vi "Read Map - Row.vi"(10 "Row":i32, 11 "map":refnum<data-value>) -> (2 "square states":T1[](array[typedef]), 3 "map":refnum<data-value>)   [LabVIEW 2020, in "DS Square.lvlib"]
uses:
  DS Square.lvlib
  Map.ctl
  Square Status.ctl
  Square State.ctl
  Center of Mass.ctl
  SubVIs/Read-Only Globals.vi
  SubVIs/Globals (private).vi
  Square/Square.lvclass
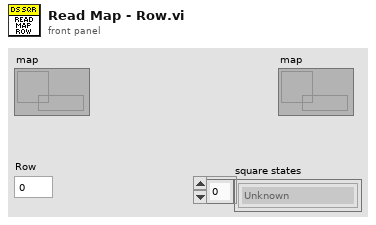
[diagram p1: front panel]
types:
  T1 = typedef "DS Square.lvlib/Square State.ctl" = enum16{"Unknown", "Empty", "Occupied - Active", "Occupied - Cool Down", "Attacked", "Enemy", "Enemy Wall"}
  T2 = typedef "DS Square.lvlib/Map.ctl" = cluster{"squares":T3[][], "center of mass":T4}
  T3 = typedef "DS Square.lvlib/Square Status.ctl" = cluster{"square state":T1, "probability":dbl, "last update":i32}
  T4 = typedef "DS Square.lvlib/Center of Mass.ctl" = cluster{"row":dbl, "col":dbl, "mass":dbl}
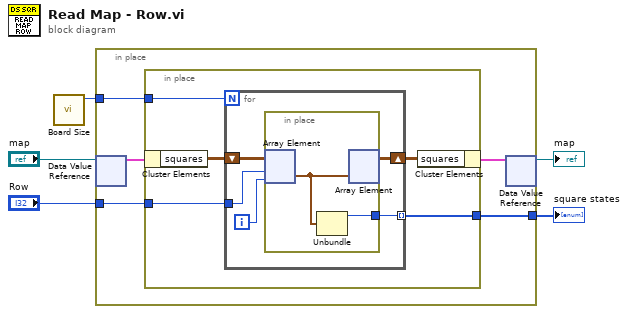
[diagram p0: block diagram]
diagram:
  n1 = call "Board Size.vi"() -> ("Board Size"=w2:i32)  [unwired: 11 in]
  n2 = in-place {
    in-place-border: "Row" -> [w10]
    in-place-border: w2 -> [w9]
    in-place-border: [w8] -> w1
    n3 = in-place-dvr #1("map") -> (w7:T2)  [unwired: 1 out]
    n4 = in-place {
      in-place-border: w10 -> [w15]
      in-place-border: w9 -> [w14]
      in-place-border: [w13] -> w8
      n5 = in-place-cluster #2(w7) -> ("squares"=w12:T3[][])
      n6 = for {
        N: w14 -> [_]
        shift-right: [w19] -> w11
        shift-left: w12 -> [w20]
        tunnel: w15 -> [w18]
        tunnel: [w16] -> w13 mode=indexing
        i -> [w17]
        n7 = in-place {
          in-place-border: [w21] -> w16
          n8 = in-place-array #3(w20, w18, w17) -> (w22:T3)
          n9 = Unbundle(w22) -> ("square state"=w21:T1)  [unwired: 2 out]
          n10 = in-place-array #3(w22) -> (w19:T3[][])  [unwired: 2 out]
        }
      }
      n11 = in-place-cluster #2("squares"=w11) -> (w6:T2)
    }
    n12 = in-place-dvr #1(w6) -> (→"map":refnum<data-value>)  [unwired: 1 out]
  }
  "square states" <- w1
